vi "Enable Switch Controller.vi"(7 "Channel (0: Channel A)":u16(ring) items=["Channel A", "Channel B"], 8 "error in (no error)":errorcluster, 9 "Enable Controller (Off)":bool, 11 "BH Druck PACE Series in":refnum<class "BH Druck PACE Series.lvclass">) -> (0 "error out":errorcluster, 3 "BH Druck PACE Series out":refnum<class "BH Druck PACE Series.lvclass">)   [LabVIEW 2022 SP3, in "BH Druck PACE Series.lvclass"]
uses:
  BH Druck PACE Series.lvclass
  BH Druck PACE Series.lvclass/BH Druck PACE Series.ctl
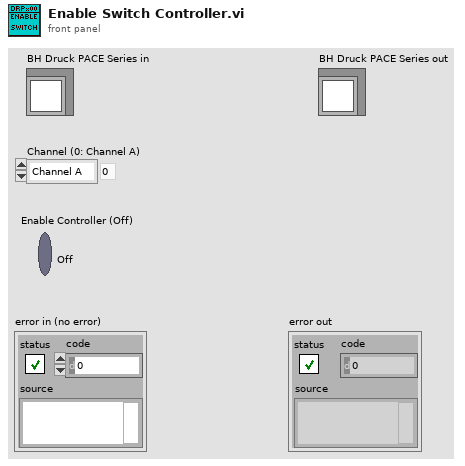
[diagram p1: front panel]
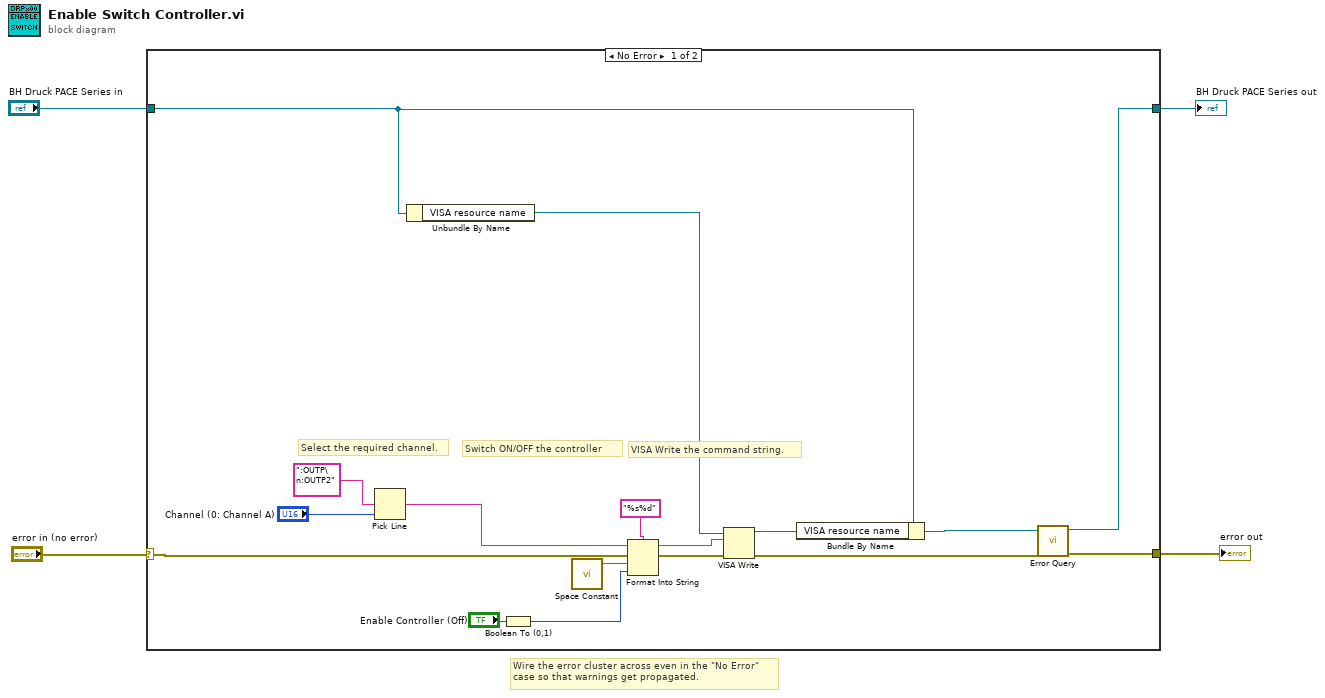
[diagram p0: block diagram]
diagram:
  # "Wire the error cluster across even in the \"No Error\"\ncase so that warnings get propagated."
  n1 = case shown="No Error" "error in (no error)" {
    selector: "error in (no error)" -> [w12 w23]
    tunnel: [w7 w23] -> w3
    tunnel: [w5 w22] -> w1
    tunnel: "BH Druck PACE Series in" -> [w10 w22]
    frame No Error {
      # "Select the required channel."
      # "Switch ON/OFF the controller"
      # "VISA Write the command string."
      n2 = Pick Line(multi-line string=":OUTP\n:OUTP2", line index="Channel (0: Channel A)") -> (output string=w18:string)  [unwired: 1 in]
      n3 = Unbundle By Name(w10) -> ("VISA resource name"=w11:refnum<visa-resource-name>)
      n4 = Boolean To (0,1)(Boolean="Enable Controller (Off)") -> (0, 1=w20:i16)
      n5 = call <vilib>:"Space Constant.vi"() -> ("String"=w21:string)
      n6 = Format Into String(format string="%s%d", initial string=w18, error in=w12, w21, w20) -> (resulting string=w16:string, error out=w17:errorcluster)
      n7 = VISA Write(VISA resource name=w11, write buffer=w16, error in (no error)=w17) -> (VISA resource name out=w9:refnum<visa-resource-name>, error out=w8:errorcluster)  [unwired: 1 out]
      n8 = Bundle By Name(cluster=w10, "VISA resource name"=w9) -> (w6:refnum<class "BH Druck PACE Series.lvclass">)
      n9 = call-dynamic "Error Query.vi"("error in (no error)"=w8, "BH Druck PACE Series in"=w6) -> ("error out"=w7:errorcluster, "BH Druck PACE Series out"=w5:refnum<class "BH Druck PACE Series.lvclass">)  [unwired: 8 in]
    }
    frame Error {
    }
  }
  "error out" <- w3
  "BH Druck PACE Series out" <- w1
